vi "LuaVIEW Pull (object).vi"(0 "kill (false)":bool, 5 "LuaVIEW reference in":T1, 11 "error in (no error)":errorcluster) -> (3 "already dead?":bool, 4 "object refnum":refnum<vi>, 6 "LuaVIEW reference out":T1, 15 "error out":errorcluster)   [LabVIEW 2013]
doc: "Retrieves an object data item from the head/bottom of the Lua stack and removes it, thereby shifting any remaining data items down by one. The returned value is a generic refnum that identifies some LabVIEW side object and must be cast to the appropriate type before use. This VI is part of a polymorphic set that supports the pulling various data types. To change the type being pulled, pop up on this VI's diagram icon and use the \"Select Type\" sub menu."
uses:
  typedefs/t_LuaVIEW Reference.ctl
  typedefs/et_LuaVIEW CIN Actions.ctl
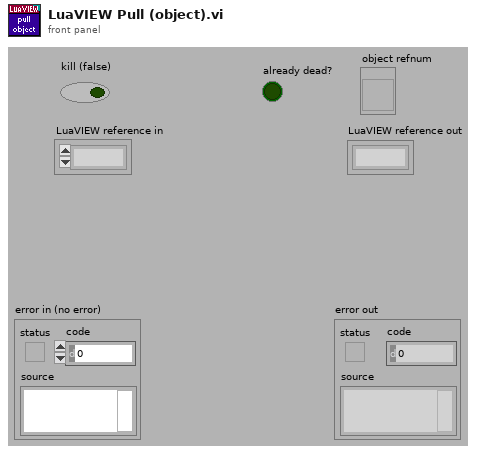
[diagram p1: front panel]
types:
  T1 = typedef "t_LuaVIEW Reference.ctl" = refnum<k1>
  T2 = typedef "et_LuaVIEW CIN Actions.ctl" = enum16{"checksynopsis", "_open", "_registerpublic", "_registerexport", "__never_an_error_result_ns", "luaversion", "cinversion", "_totals", "_taskcount", "pathological", "_unregnextpublic", "registryusecount", "__per_state_actions", "regsetprivate", "regsetindex", "regsetmodule", "_revokeexports", "_usepublic", "prepare", "compile", "execute", "call", "unregstaterefs", "_close", "pullboolean", "pullnumber", "pullI8", "pullU8", "pullI16", "pullU16", "pullI32", "pullU32", "pullobject", "pullrefnum", "pullstring", "pullflat", "pushflat", "pushobject", "getattribute", "setattribute", "stacktostring", "_startyieldtest", "_endyieldtest", "_pollprintbuffer", "__never_an_error_result_ps", "_pollexport", "setclone", "forcecleanup", "gettop", "clearstack", "insert", "pushboolean", "pushnumber", "pushrefnum", "pushstring", "pushnil", "pushvalue", "gettaskref", "settaskref"}
  T3 = typedef "et_LuaVIEW CIN Results.ctl" = enum16{"OK", "error", "main", "call", "clonecall", "modulecall", "exportcall", "index", "yield"}
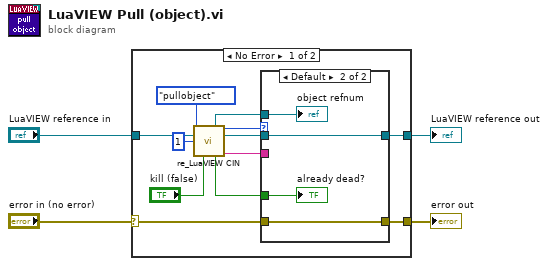
[diagram p0: block diagram]
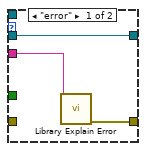
[diagram p2: hidden frame]
diagram:
  n1 = case shown="No Error" "error in (no error)" {
    selector: "error in (no error)" -> [w7 w25]
    tunnel: [w12 w24] -> w4
    tunnel: [w9 w25] -> w3
    tunnel: "LuaVIEW reference in" -> [w15 w24]
    frame No Error {
      n2 = call "re_LuaVIEW CIN.vi"("action"=et_LuaVIEW_CIN_Actions."pullobject", "LuaVIEW reference in"=w15, "index in"=1, "boolean in"="kill (false)") -> ("refnum out"=w11:refnum<vi>, "result"=w10:T3, "LuaVIEW reference out"=w13:T1, "boolean out"=w5:bool, "string out"=w8:string)  [unwired: 5 in, 2 out]
      n3 = case shown="Default" w10 {
        tunnel: w13 -> [w17 w20]
        tunnel: [w17 w20] -> w12
        tunnel: w11 -> [_ w23]
        tunnel: [w19 w22] -> w9
        tunnel: w8 -> [w18 _]
        tunnel: w7 -> [_ w22]
        tunnel: w5 -> [_ w21]
        frame "error" {
          n4 = call "Library Explain Error.vi"("explanation prefix (none)"=w18) -> ("explained error"=w19:errorcluster)  [unwired: 14 in]
        }
        frame Default {
          "object refnum" <- w23
          "already dead?" <- w21
        }
      }
    }
    frame Error {
    }
  }
  "LuaVIEW reference out" <- w4
  "error out" <- w3
